vi "MeasureRMS(SubVI).vi"(10 "Sampling Rate (Hz)":dbl, 11 "# of samples":i32) -> (2 "AC estimate (Vrms)":dbl, 3 "data":dynamicdata(waveform))   [LabVIEW 2015]
uses:
  <vilib>/Analysis/NI_AALPro.lvlib
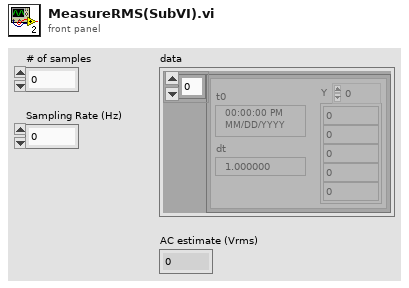
[diagram p1: front panel]
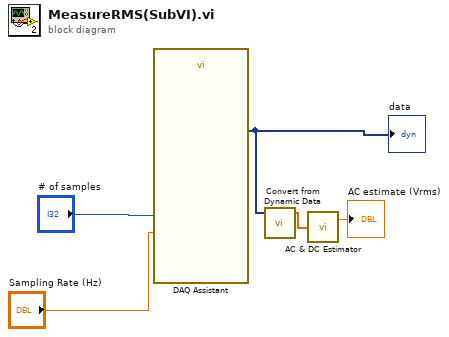
[diagram p0: block diagram]
diagram:
  n1 = call "DAQ Assistant"("rate"="Sampling Rate (Hz)", "number of samples"="# of samples") -> ("data"=w4:dynamicdata)  [unwired: 15 in, 2 out]
  "data" <- w4
  n2 = call "Convert from Dynamic Data"("Dynamic Data Type"=w4) -> ("Array"=w1:dbl[])  [unwired: 3 in]
  n3 = call <vilib>:"AC & DC Estimator.vi"("Signal (V)"=w1) -> ("AC estimate (Vrms)"=→"AC estimate (Vrms)":dbl)  [unwired: 1 out]
